vi "Setting Database.NewCurrentPath.vi"(8 "error in (no error)":errorcluster, 10 "NewCurrentPath":T1, 11 "Setting Database":refnum<class "Setting Database.lvclass">) -> (0 "error out":errorcluster, 3 "Setting Database out":refnum<class "Setting Database.lvclass">)   [LabVIEW 2020, in "Setting Database.lvclass"]
doc: "---------------------------------------------------------------\nJKI State Machine Objects™\nhttp://jki.net/state-machine-objects/\nCopyright (C) 2005-2015, JKI <info@jki.net>\nALL RIGHTS RESERVEDJKI State Machine Objects (SMO) 1.0.0.4\nJKI - JKI\nCopyright (c) 2015, JKI"
uses:
  Setting Database.lvclass
  Typedefs/PublicEvents--Setting Database.NewCurrentPath.ctl
  Setting Database.lvclass/Setting Database.ctl
  Path Settings/Path Settings.lvclass
panel:
  # "For instructions on how to use the JKI State Machine Objects, examples and video tutorials, visit:\nhttp://jki.net/state-machine-objects/\n\nJKI State Machine Objects™\nhttp://jki.net/state-machine-objects/\nCopyright (C) 2005-2015, JKI <info@jki.net>\nALL RIGHTS RESERVED"
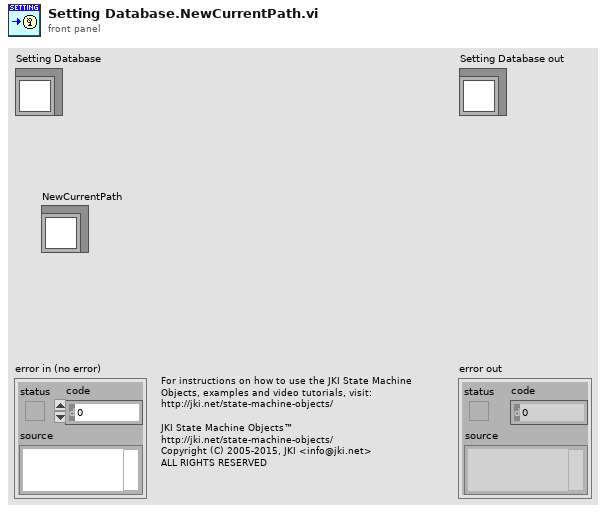
[diagram p1: front panel]
types:
  T1 = typedef "Setting Database.lvclass/PublicEvents--Setting Database.NewCurrentPath.ctl" = refnum<class "Path Settings.lvclass">
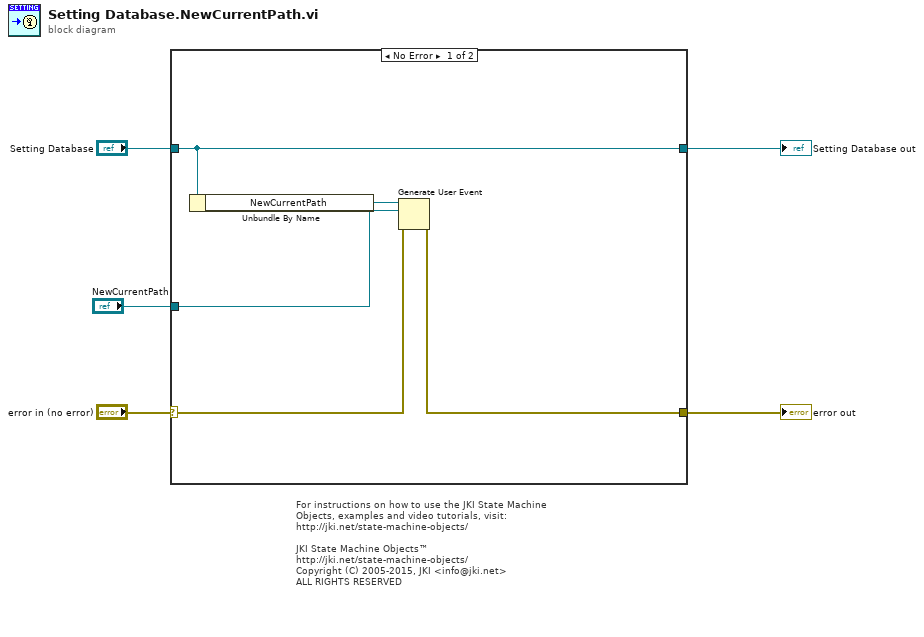
[diagram p0: block diagram]
diagram:
  # "For instructions on how to use the JKI State Machine Objects, examples and video tutorials, visit:\nhttp://jki.net/state-machine-objects/\n\nJKI State Machine Objects™\nhttp://jki.net/state-machine-objects/\nCopyright (C) 2005-2015, JKI <info@jki.net>\nALL RIGHTS RESERVED"
  n1 = case shown="No Error" "error in (no error)" {
    selector: "error in (no error)" -> [w10 w12]
    tunnel: [w7 w12] -> w4
    tunnel: [w6 w11] -> w5
    tunnel: "Setting Database" -> [w6 w11]
    tunnel: "NewCurrentPath" -> [w9 _]
    frame No Error {
      n2 = Unbundle By Name(w6) -> ("NewCurrentPath"=w8:refnum<user-event>)
      n3 = Generate User Event(user event=w8, event data cluster=w9, error in=w10) -> (error out=w7:errorcluster)  [unwired: 1 in, 1 out]
    }
    frame Error {
    }
  }
  "error out" <- w4
  "Setting Database out" <- w5
